vi "tiffTags.vi"(8 "error in (no error)":errorcluster, 9 "tif pointer":i64) -> (0 "error out":errorcluster, 1 "tiff pointer":i64, 3 "Image Properties":T1)   [LabVIEW 2013]
uses:
  tags_cluster.ctl
  imagereconstruction/x64/Debug/labviewdll.dll
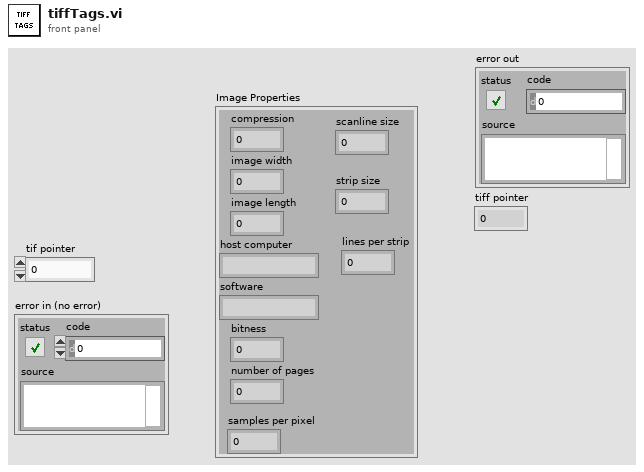
[diagram p1: front panel]
types:
  T1 = typedef "tags_cluster.ctl" = cluster{"compression":i32, "image width":i32, "image length":i32, "host computer":string, "software":string, "bitness":i32, "number of pages":i32, "samples per pixel":i32, "scanline size":i32, "strip size":i32, "lines per strip":i32}
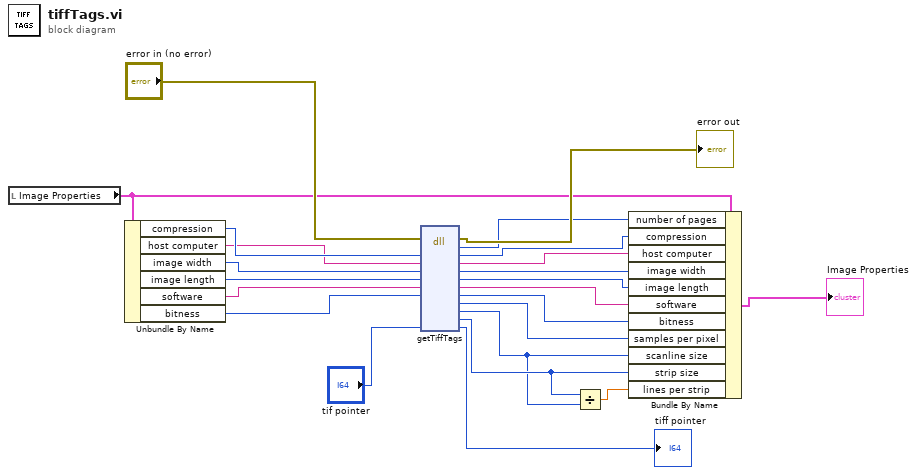
[diagram p0: block diagram]
diagram:
  n1 = local read "Image Properties"() -> (w11:T1)
  n2 = Unbundle By Name(w11) -> ("compression"=w10:i32, "host computer"=w9:string, "image width"=w8:i32, "image length"=w7:i32, "software"=w6:string, "bitness"=w5:i32)
  n3 = dll-call lib="D:/work/uni/FYP/reconrepo/imagereconstruction/x64/Debug/labviewdll.dll" fn="getTiffTags"(error in="error in (no error)", "compression"=w10, "host computer"=w9, "imageWidth"=w8, "imageLength"=w7, "software"=w6, "bitness"=w5, "tiff pointer"="tif pointer") -> (error out=→"error out":errorcluster, "number of pages"=w13:u32, "compression"=w22:i32, "host computer"=w21:string, "imageWidth"=w20:i32, "imageLength"=w17:i32, "software"=w18:string, "bitness"=w16:i32, "samples per pixel"=w4:i32, "scanline size"=w2:i32, "strip size"=w3:i32, "tiff pointer"=→"tiff pointer":i64)  [unwired: 5 in, 1 out]
  n4 = Divide(x=w3, y=w2) -> (x/y=w1:dbl)
  n5 = Bundle By Name(cluster=w11, "number of pages"=w13, "compression"=w22, "host computer"=w21, "image width"=w20, "image length"=w17, "software"=w18, "bitness"=w16, "samples per pixel"=w4, "scanline size"=w2, "strip size"=w3, "lines per strip"=w1) -> (→"Image Properties":T1)
